vi "Lockin.DAQ.Create.vi"(8 "error in":errorcluster, 11 "Instrument.DAQ":refnum<class "Instrument.DAQ.lvclass">) -> (0 "error out":errorcluster, 3 "Instrument.DAQ":refnum<class "Instrument.DAQ.lvclass">)   [LabVIEW 2019, in "Instrument.DAQ.lvclass"]
uses:
  Instrument.DAQ.lvclass
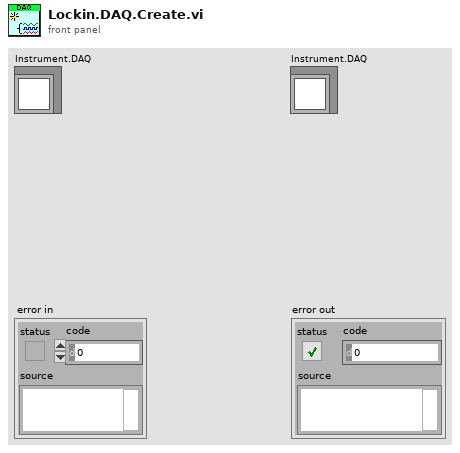
[diagram p1: front panel]
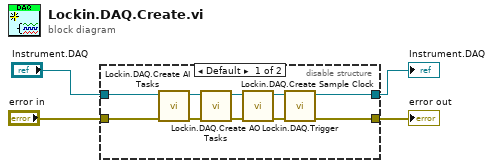
[diagram p0: block diagram]
diagram:
  n1 = disable-structure shown="Default" {
    disable-tunnel: "Instrument.DAQ" -> [w8 w16]
    disable-tunnel: "error in" -> [w7 w15]
    disable-tunnel: [w6 w16] -> w3
    disable-tunnel: [w5 w15] -> w2
    frame condition #0 (active) {
      n2 = call "Lockin.DAQ.Create AI Tasks.vi"("error in"=w7, "Instrument.DAQ"=w8) -> ("error out"=w9:errorcluster, "Instrument.DAQ"=w10:refnum<class "Instrument.DAQ.lvclass">)  [unwired: 8 in]
      n3 = call "Lockin.DAQ.Create AO Tasks.vi"("error in (no error)"=w9, "Instrument.DAQ"=w10) -> ("error out"=w11:errorcluster, "Instrument.DAQ"=w12:refnum<class "Instrument.DAQ.lvclass">)  [unwired: 8 in]
      n4 = call "Lockin.DAQ.Create Sample Clock.vi"("error in (no error)"=w11, "Instrument.DAQ"=w12) -> ("error out"=w13:errorcluster, "Instrument.DAQ"=w14:refnum<class "Instrument.DAQ.lvclass">)  [unwired: 8 in]
      n5 = call "Lockin.DAQ.Trigger.vi"("error in (no error)"=w13, "Instrument.DAQ"=w14) -> ("error out"=w5:errorcluster, "Instrument.DAQ"=w6:refnum<class "Instrument.DAQ.lvclass">)  [unwired: 8 in]
    }
    frame condition #1 {
    }
  }
  "error out" <- w2
  "Instrument.DAQ" <- w3
